vi "WriteToCVT.vi"(4 "non compressed string":string, 6 "compressed string":string, 7 "force CVT update":bool, 8 "error in":errorcluster, 9 "non compressed":bool, 10 "compressed":bool, 11 "variable":string) -> (0 "error out":errorcluster)   [LabVIEW 2011]
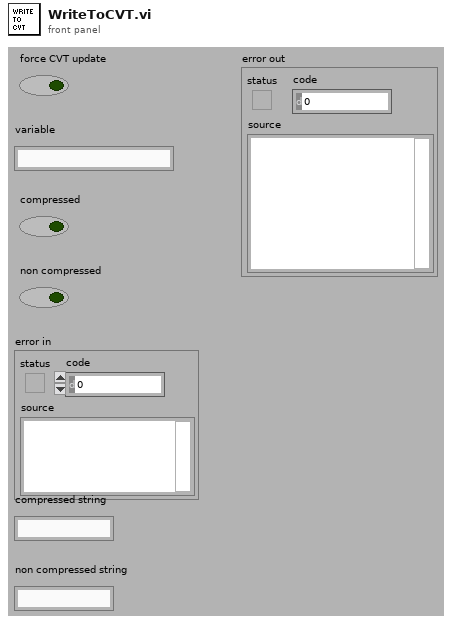
[diagram p1: front panel]
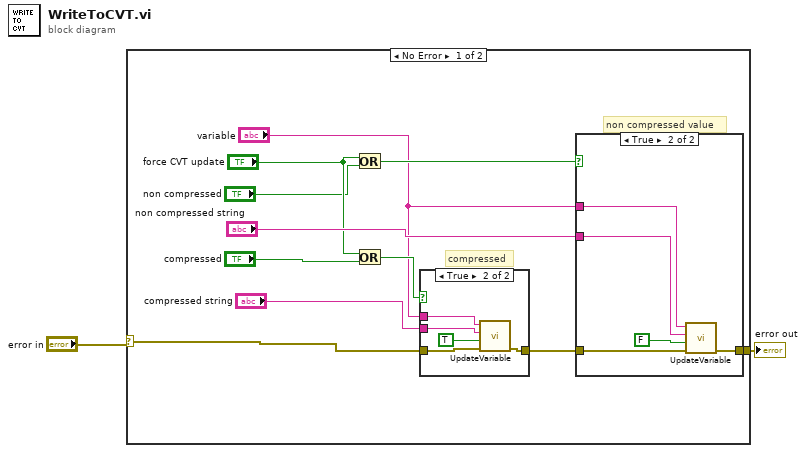
[diagram p0: block diagram]
diagram:
  n1 = case shown="No Error" "error in" {
    selector: "error in" -> [w3 w26]
    tunnel: [w4 w26] -> w2
    frame No Error {
      # "compressed"
      # "non compressed value"
      n2 = Or(x="force CVT update", y="non compressed") -> (x .or. y?=w12:bool)
      n3 = Or(x="force CVT update", y="compressed") -> (x .or. y?=w11:bool)
      n4 = case shown="True" w11 {
        tunnel: w3 -> [w14 w19]
        tunnel: [w14 w18] -> w5
        tunnel: "compressed string" -> [_ w16]
        tunnel: "variable" -> [_ w15]
        frame False {
        }
        frame True {
          n5 = call "UpdateVariable.vi"("error in"=w19, "compressed"=TRUE, "value in"=w16, "variable"=w15) -> ("error out"=w18:errorcluster)  [unwired: 7 in]
        }
      }
      n6 = case shown="True" w12 {
        tunnel: w5 -> [w20 w25]
        tunnel: [w20 w24] -> w4
        tunnel: "non compressed string" -> [_ w22]
        tunnel: "variable" -> [_ w21]
        frame False {
        }
        frame True {
          n7 = call "UpdateVariable.vi"("error in"=w25, "compressed"=FALSE, "value in"=w22, "variable"=w21) -> ("error out"=w24:errorcluster)  [unwired: 7 in]
        }
      }
    }
    frame Error {
    }
  }
  "error out" <- w2
